vi "uint32_wrapSubtract.vi"() -> ()   [LabVIEW 2013]
panel:
  out "Numeric":u32
  in  "Curr (ms)":u32
  in  "Tick count (ms)":u32
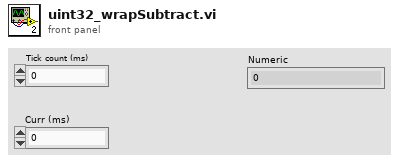
[diagram p1: front panel]
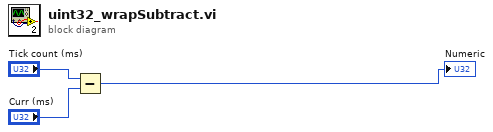
[diagram p0: block diagram]
diagram:
  n1 = Subtract(x="Tick count (ms)", y="Curr (ms)") -> (x-y=→"Numeric":u32)
